vi "Configure Cascade Outer Loop PID Set.vi"(0 "VISA resource name":refnum<visa-resource-name>, 1 "Set (1)":i16=1, 2 "Channels (0: 1A)":i16(ring) items=["1A", "1B"], 3 "Proportional Band (25.0)":dbl=25.0 format="%.2f", 4 "Integral/Reset (0.0)":dbl format="%.2f", 5 "error in (no error)":errorcluster {"code" format="%.0x"}, 6 "Unit Address (1)":i16=1, 8 "Derivative/Rate (0.0)":dbl format="%.2f", 10 "Dead Band (0.0)":dbl format="%.2f", 12 "Hysteresis (3.0)":dbl=3.0 format="%.2f") -> (14 "VISA resource name out":refnum<visa-resource-name>, 19 "error out":errorcluster {"code" format="%.0x"})   [LabVIEW 2010]
doc: "This VI configures cascade outer loop PID sets."
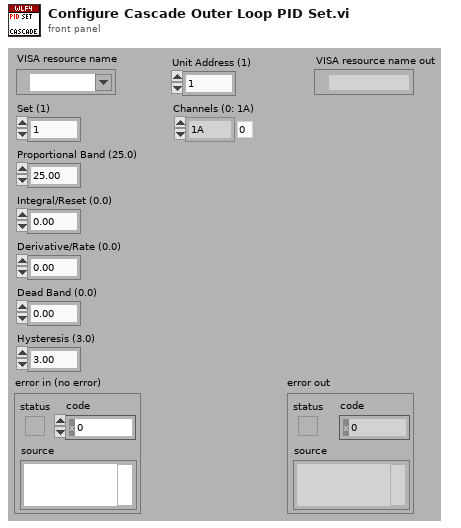
[diagram p1: front panel]
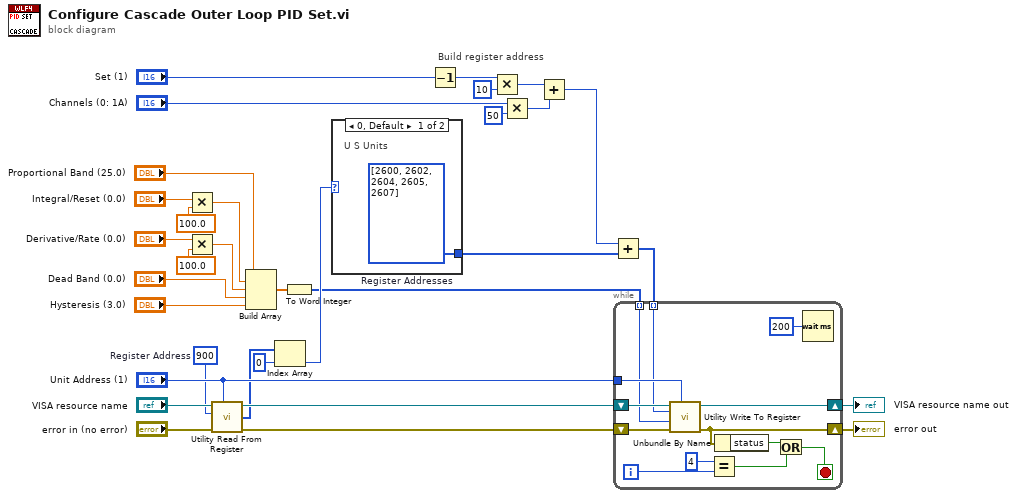
[diagram p0: block diagram]
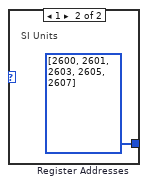
[diagram p2: hidden frame]
diagram:
  w22 = u16 900  # Register Address
  # "Build register address"
  n1 = Multiply(x="Integral/Reset (0.0)", y=100.0) -> (x*y=w9:dbl)
  n2 = Multiply(x="Derivative/Rate (0.0)", y=100.0) -> (x*y=w14:dbl)
  n3 = call "Utility Read From Register.vi"("Unit Address (1)"="Unit Address (1)", "error in (no error)"="error in (no error)", "Register Address (0)"=w22, "VISA resource name"="VISA resource name") -> ("error out"=w26:errorcluster, "Data"=w20:i16[], "VISA resource name out"=w25:refnum<visa-resource-name>)  [unwired: 5 in]
  n4 = Build Array("Proportional Band (25.0)", w9, w14, "Dead Band (0.0)", "Hysteresis (3.0)") -> (w11:dbl[])
  n5 = Index Array(array=w20, index=0) -> (element=w19:i16)
  n6 = To Word Integer(number=w11) -> (16bit integer=w1:i16[])
  n7 = case shown="0, Default" w19 {
    tunnel: [w33 w34] -> w18
    frame 0, Default {
      w33 = i32[] [2600, 2602, 2604, 2605, 2607]  # Register Addresses
      # "U S Units"
    }
    frame 1 {
      w34 = i32[] [2600, 2601, 2603, 2605, 2607]  # Register Addresses
      # "SI Units"
    }
  }
  n8 = Decrement(x="Set (1)") -> (x-1=w6:i16)
  n9 = Multiply(x=w6, y=i16 10) -> (x*y=w4:i16)
  n10 = Multiply(x="Channels (0: 1A)", y=i16 50) -> (x*y=w3:i16)
  n11 = Add(x=w4, y=w3) -> (x+y=w2:i16)
  n12 = Add(x=w2, y=w18) -> (x+y=w29:i32[])
  n13 = while {
    tunnel: "Unit Address (1)" -> [w47]
    shift-right: [w44] -> w32
    shift-left: w25 -> [w46]
    shift-right: [w41] -> w31
    shift-left: w26 -> [w45]
    tunnel: w29 -> [w42] mode=indexing
    tunnel: w1 -> [w35] mode=indexing
    i -> [w38]
    stop <- w39 stop-if-true
    n14 = call "Utility Write To Register.vi"("Unit Address (1)"=w47, "error in (no error)"=w45, "Data (0)"=w35, "Register Address (0)"=w42, "VISA resource name"=w46) -> ("error out"=w41:errorcluster, "VISA resource name out"=w44:refnum<visa-resource-name>)  [unwired: 5 in]
    n15 = Equal?(x=4, y=w38) -> (x = y?=w36:bool)
    n16 = Unbundle By Name(w41) -> ("status"=w40:bool)
    n17 = Or(x=w40, y=w36) -> (x .or. y?=w39:bool)
    n18 = Wait (ms)(milliseconds to wait=u32 200) -> ()  [unwired: 1 out]
  }
  "error out" <- w31
  "VISA resource name out" <- w32
